vi "XML - Create XML file.vi"(8 "error in (no error)":errorcluster, 10 "Consolidated_CD":refnum<class "NIVS_Consolidated_CDW_MetaDataObj.lvclass">, 11 "CD Wizard - Internal Data":T1) -> (0 "error out":errorcluster)   [LabVIEW 2019, in "NIVS_Consolidated_CDW_MetaDataObj.lvclass"]
doc: "Create the XML file and alter the content of the file, so that it fits for the generated custom device."
uses:
  NIVS_Consolidated_CDW_MetaDataObj.lvclass
  Internal data.ctl
  C:/Program Files (x86)/National Instruments/LabVIEW 2019/resource/dialog/NewProjectWizard/MetaDataObj/MetaDataObj.lvclass
  Create XML-file - States.ctl
  <resource>/dialog/NewProjectWizard/MetaDataObj/MetaDataObj.lvclass/MetaDataObj.ctl
  NIVS_Consolidated_CDW_MetaDataObj.lvclass/NIVS_Consolidated_CDW_MetaDataObj.ctl
  Template Classes/NIVS_CD Template/NIVS_CD Template.lvclass/NIVS_CD Template.ctl
  CD System Explorer lvlib.ctl
  Target Type.ctl
  Template Classes/NIVS_CD Template/Read Submenu.vi
  Template Classes/NIVS_CD Template/Read Parent Menu.vi
  Template Classes/NIVS_CD Template/Read Max Instances.vi
  <resource>/dialog/NewProjectWizard/MetaDataObj/Accessors/Read Project Root.vi
  <resource>/dialog/NewProjectWizard/MetaDataObj/Accessors/Read Project Name.vi
  Read CD Template.vi
  CD System Explorer lvlib.vi
  Template Classes/NIVS_CD Template/NIVS_CD Template.lvclass
  <vilib>/Utility/Data Type/NI_Data Type.lvlib
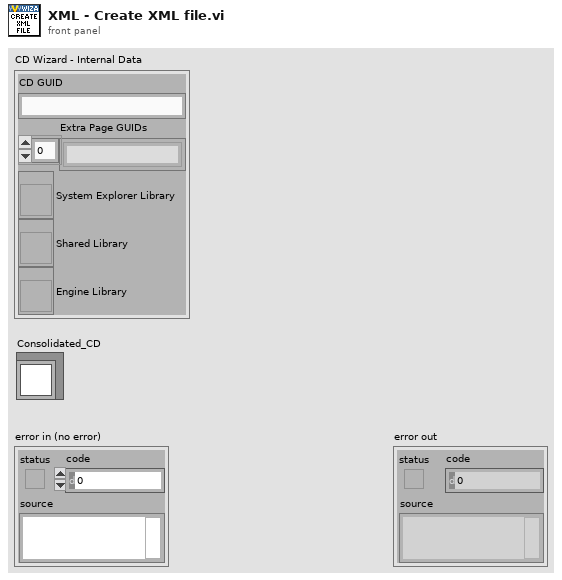
[diagram p1: front panel]
types:
  T1 = typedef "NIVS_Consolidated_CDW_MetaDataObj.lvclass/Internal data.ctl" = cluster{"CD GUID":string, "Extra Page GUIDs":string[], "System Explorer Library":refnum<vi>, "Shared Library":refnum<vi>, "Engine Library":refnum<vi>}
  T2 = typedef "NIVS_Consolidated_CDW_MetaDataObj.lvclass/Create XML-file - States.ctl" = enum16{"Read XML template file", "Change CD -MenuName-", "Change CD -Name-", "Change CD -Type-", "Change CD -Occurrences-", "Change CD -MainPageGUID-", "Change CD -InitVIPath-", "Change CD -WindowsCustomDeviceVIPath-", "Change CD -WindowsCustomDeviceVIRTPath-", "Change CD -PharlapCustomDeviceVIPath-", "Change CD -PharlapCustomDeviceVIRTPath-", "Change CD -VxWorksCustomDeviceVIPath-", "Change CD -VxWorksCustomDeviceVIRTPath-", "Change CD -LinuxARMCustomDeviceVIPath-", "Change CD -LinuxARMCustomDeviceVIRTPath-", "Change CD -Linuxx64CustomDeviceVIPath-", "Change CD -Linuxx64CustomDeviceVIRTPath-", "Change CD -MainPageVIPath-", "Change CD -ExtraPages-", "Change CD -ActionVIOnCompile-", "Change CD -ExportConfigurationRTM-", "Write XML file content back"}
  T3 = typedef "NIVS_Consolidated_CDW_MetaDataObj.lvclass/CD System Explorer lvlib.ctl" = enum16{"LibraryFileName", "LibraryFolderName", "System Explorer.FolderName", "System Explorer.Dynamically Called.FolderName", "System Explorer.Dynamically Called.Extra Pages.FolderName", "System Explorer.Dynamically Called.Extra Pages.TemplatePathAndName", "System Explorer.Dynamically Called.Main Page.VIName", "System Explorer.Dynamically Called.Main Page.TemplatePathAndName", "System Explorer.Dynamically Called.Initialization VI.VIName", "System Explorer.Dynamically Called.Initialization VI.TemplatePathAndName", "System Explorer.SubVI.FolderName", "System Explorer.Types.FolderName", "System Explorer.ActionVIOnCompile.VIName", "System Explorer.ExportConfigRTM.VIName", "System Explorer.LoadHelpFile.VIName"}
  T4 = typedef "NIVS_Consolidated_CDW_MetaDataObj.lvclass/Target Type.ctl" = enum16{"Windows", "VxWorks", "Pharlap", "Linux 32 ARM", "Linux x64"}
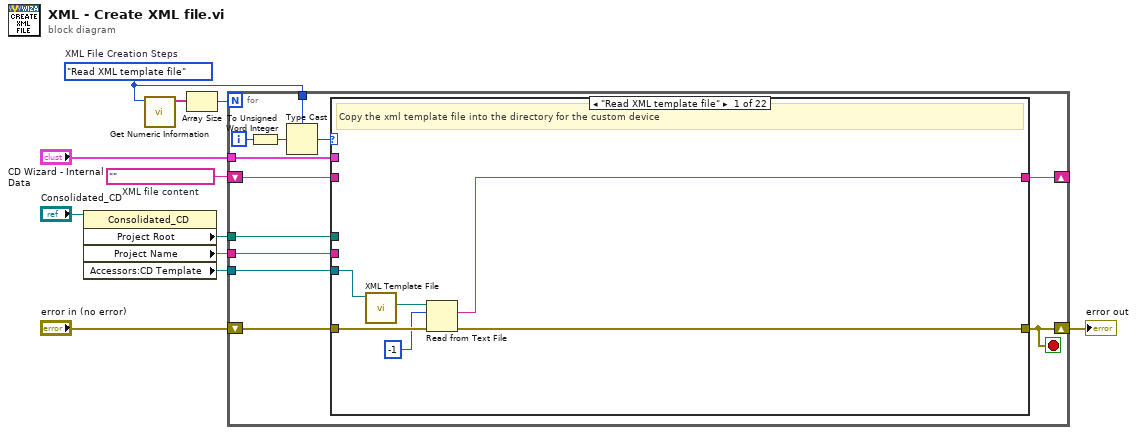
[diagram p0: block diagram]
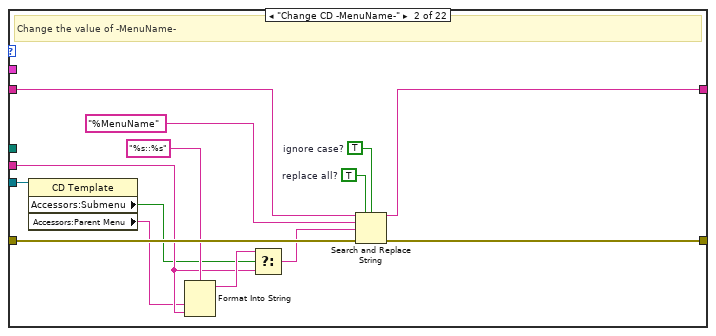
[diagram p2: hidden frame]
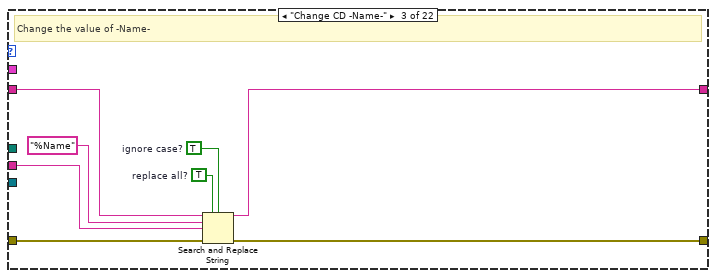
[diagram p3: hidden frame]
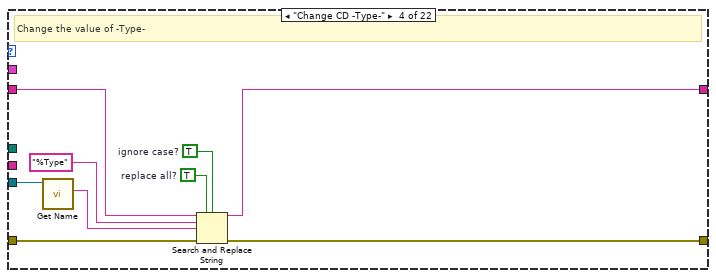
[diagram p4: hidden frame]
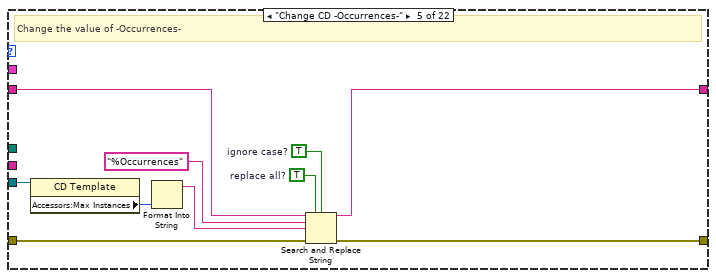
[diagram p5: hidden frame]
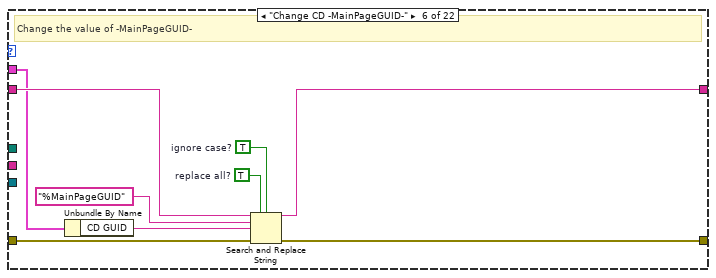
[diagram p6: hidden frame]
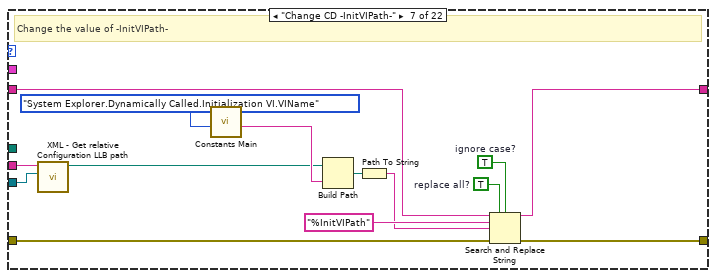
[diagram p7: hidden frame]
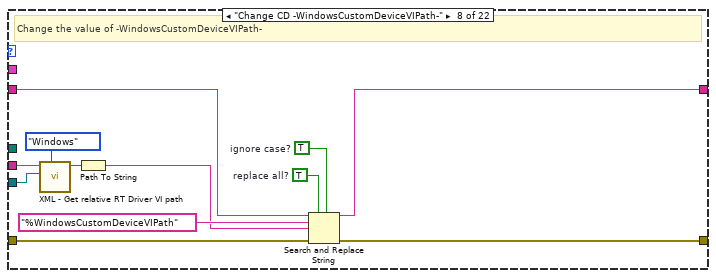
[diagram p8: hidden frame]
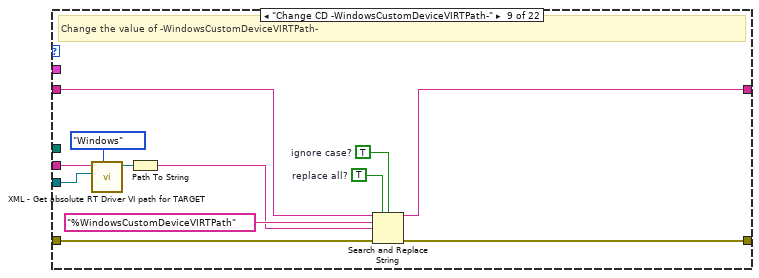
[diagram p9: hidden frame]
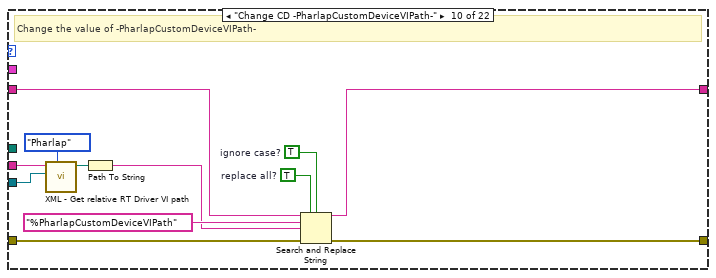
[diagram p10: hidden frame]
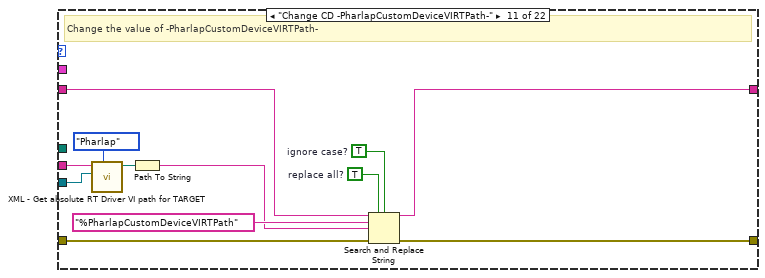
[diagram p11: hidden frame]
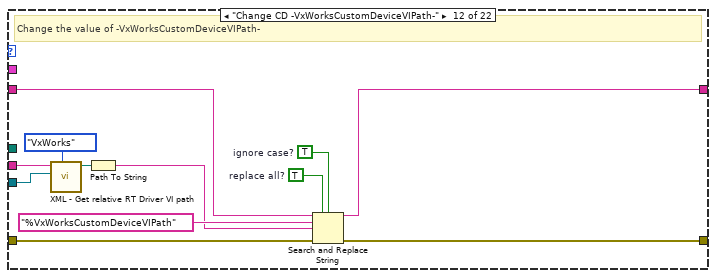
[diagram p12: hidden frame]
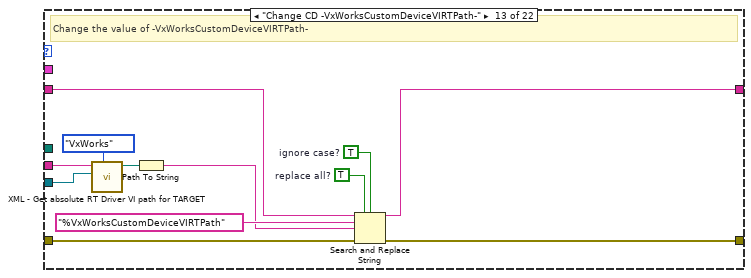
[diagram p13: hidden frame]
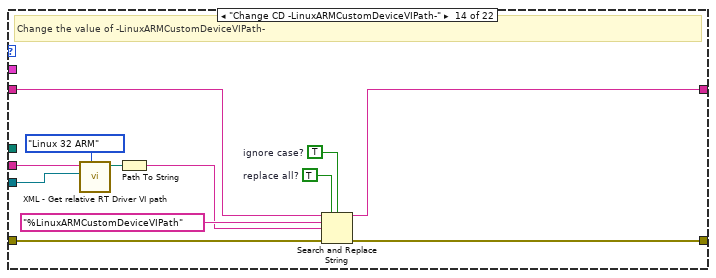
[diagram p14: hidden frame]
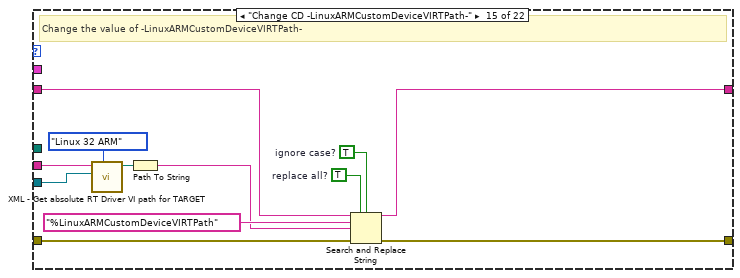
[diagram p15: hidden frame]
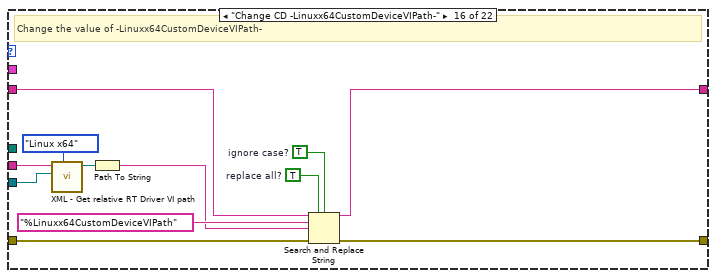
[diagram p16: hidden frame]
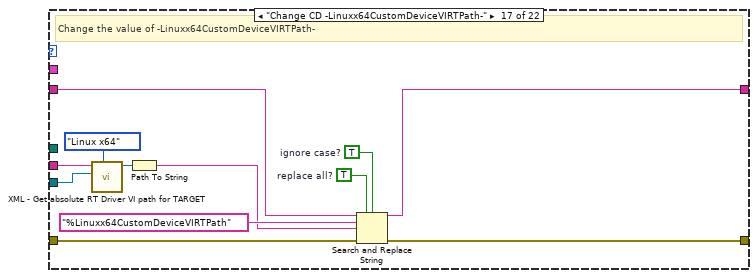
[diagram p17: hidden frame]
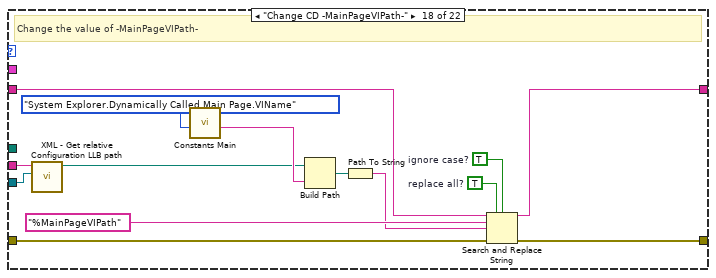
[diagram p18: hidden frame]
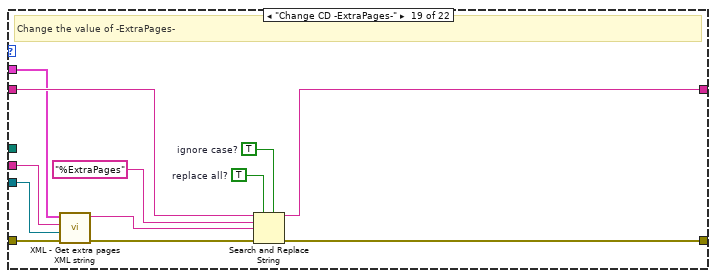
[diagram p19: hidden frame]
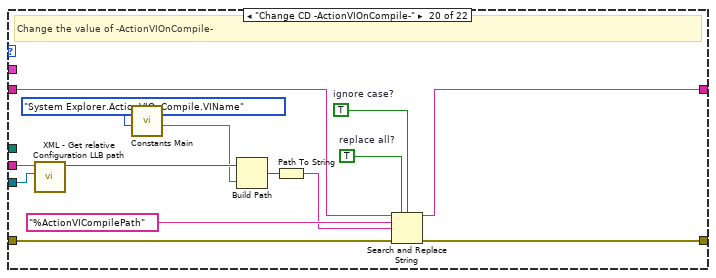
[diagram p20: hidden frame]
diagram:
  w2 = Create_XML-file_-_States."Read XML template file"  # XML File Creation Steps
  w10 = ""  # XML file content
  n1 = property class="Consolidated_CD"(reference="Consolidated_CD") -> ("Project Root"=w8:path, "Project Name"=w7:string, "Accessors:CD Template"=w6:refnum<class "NIVS_CD Template.lvclass">)  [unwired: 1 in, 2 out]
  n2 = call <vilib>:"Get Numeric Information.vi"("variant"=w2) -> ("enum names"=w3:string[])  [unwired: 7 in, 3 out]
  n3 = Array Size(array=w3) -> (size(s)=w4:i32)
  n4 = for {
    N: w4 -> [_]
    shift-right: [w18] -> w11
    shift-left: "error in (no error)" -> [w17]
    shift-right: [w22] -> _
    shift-left: w10 -> [w23]
    tunnel: w8 -> [w21]
    tunnel: w7 -> [w20]
    tunnel: w6 -> [w19]
    tunnel: w2 -> [w15]
    tunnel: "CD Wizard - Internal Data" -> [w12]
    i -> [w16]
    stop <- w18 stop-if-true
    # "While loop for State Machine"
    n5 = To Unsigned Word Integer(number=w16) -> (unsigned 16bit integer=w14:u16)
    n6 = Type Cast(type=w15, x=w14) -> (*(type *) &x=w13:T2)
    n7 = case shown="\"Read XML template file\"" w13 {
      tunnel: w17 -> [w27 w39 w47 w54 w61 w72 w82 w96 w108 w120 w132 w144 w156 w168 w180 w192 w204 w216 w230 w240 w254 w277]
      tunnel: [w28 w40 w48 w57 w67 w76 w90 w104 w115 w127 w139 w151 w163 w175 w187 w199 w211 w224 w236 w250 w257 w280] -> w18
      tunnel: w12 -> [_ _ _ _ _ w75 _ _ _ _ _ _ _ _ _ _ _ _ w234 _ _ _]
      tunnel: w23 -> [_ w42 w50 w59 w69 w78 w92 w101 w117 w129 w141 w153 w165 w177 w189 w201 w213 w226 w238 w252 w271 w279]
      tunnel: [w24 w41 w49 w58 w68 w77 w91 w105 w116 w128 w140 w152 w164 w176 w188 w200 w212 w225 w237 w251 w261 w279] -> w22
      tunnel: w21 -> [_ _ _ _ _ _ _ _ _ _ _ _ _ _ _ _ _ _ _ _ _ w276]
      tunnel: w20 -> [_ w33 w44 _ _ _ w81 w95 w107 w119 w131 w143 w155 w167 w179 w191 w203 w215 w229 w242 w256 w275]
      tunnel: w19 -> [w29 w32 _ w53 w63 _ w80 w94 w106 w118 w130 w142 w154 w166 w178 w190 w202 w214 w228 w241 w255 w274]
      frame "Read XML template file" {
        # "Copy the xml template file into the directory for the custom device"
        n8 = call-dynamic "XML Template File.vi"("CD Template"=w29) -> ("XML Template File"=w26:path)  [unwired: 10 in]
        n9 = Read from Text File(file (use dialog)=w26, count=-1, error in=w27) -> (text=w24:string, error out=w28:errorcluster)  [unwired: 1 in, 2 out]
      }
      frame "Change CD -MenuName-" {
        w37 = TRUE  # ignore case?
        w38 = TRUE  # replace all?
        # "Change the value of -MenuName-"
        n10 = property class="CD Template"(reference=w32) -> ("Accessors:Submenu"=w31:bool, "Accessors:Parent Menu"=w30:string)  [unwired: 1 in, 2 out]
        n11 = Format Into String(format string="%s::%s", w30, w33) -> (resulting string=w35:string)  [unwired: 2 in, 1 out]
        n12 = Select(t=w35, s=w31, f=w33) -> (s? t:f=w34:string)
        n13 = Search and Replace String(replace all?=w38, case sensitive?=w37, input string=w42, search string="%MenuName", replace string=w34, error in=w39) -> (result string=w41:string, error out=w40:errorcluster)  [unwired: 1 in, 3 out]
      }
      frame "Change CD -Name-" {
        w45 = TRUE  # ignore case?
        w46 = TRUE  # replace all?
        # "Change the value of -Name-"
        n14 = Search and Replace String(replace all?=w46, case sensitive?=w45, input string=w50, search string="%Name", replace string=w44, error in=w47) -> (result string=w49:string, error out=w48:errorcluster)  [unwired: 1 in, 3 out]
      }
      frame "Change CD -Type-" {
        w55 = TRUE  # ignore case?
        w56 = TRUE  # replace all?
        # "Change the value of -Type-"
        n15 = call-dynamic "Get Name.vi"("CD Template"=w53) -> ("String"=w52:string)  [unwired: 10 in]
        n16 = Search and Replace String(replace all?=w56, case sensitive?=w55, input string=w59, search string="%Type", replace string=w52, error in=w54) -> (result string=w58:string, error out=w57:errorcluster)  [unwired: 1 in, 3 out]
      }
      frame "Change CD -Occurrences-" {
        w64 = TRUE  # ignore case?
        w66 = TRUE  # replace all?
        # "Change the value of -Occurrences-"
        n17 = property class="CD Template"(reference=w63) -> ("Accessors:Max Instances"=w62:u32)  [unwired: 1 in, 2 out]
        n18 = Format Into String(w62) -> (resulting string=w65:string)  [unwired: 3 in, 1 out]
        n19 = Search and Replace String(replace all?=w66, case sensitive?=w64, input string=w69, search string="%Occurrences", replace string=w65, error in=w61) -> (result string=w68:string, error out=w67:errorcluster)  [unwired: 1 in, 3 out]
      }
      frame "Change CD -MainPageGUID-" {
        w71 = TRUE  # ignore case?
        w74 = TRUE  # replace all?
        # "Change the value of -MainPageGUID-"
        n20 = Unbundle By Name(w75) -> ("CD GUID"=w73:string)
        n21 = Search and Replace String(replace all?=w74, case sensitive?=w71, input string=w78, search string="%MainPageGUID", replace string=w73, error in=w72) -> (result string=w77:string, error out=w76:errorcluster)  [unwired: 1 in, 3 out]
      }
      frame "Change CD -InitVIPath-" {
        w88 = TRUE  # ignore case?
        w89 = TRUE  # replace all?
        # "Change the value of -InitVIPath-"
        n22 = call "XML - Get relative Configuration LLB path.vi"("CD Template"=w80, "Project Name"=w81) -> ("Relative Configuration LLB path"=w83:path)  [unwired: 9 in]
        n23 = call-poly "Constants Main.vi"("Action"=CD_System_Explorer_lvlib."System Explorer.Dynamically Called.Initialization VI.VIName") -> ("Output"=w86:string)  [unwired: 10 in]
        n24 = Build Path(base path=w83, name or relative path=w86) -> (appended path=w84:path)
        n25 = Path To String(path=w84) -> (string=w87:string)
        n26 = Search and Replace String(replace all?=w89, case sensitive?=w88, input string=w92, search string="%InitVIPath", replace string=w87, error in=w82) -> (result string=w91:string, error out=w90:errorcluster)  [unwired: 1 in, 3 out]
      }
      frame "Change CD -WindowsCustomDeviceVIPath-" {
        w102 = TRUE  # ignore case?
        w103 = TRUE  # replace all?
        # "Change the value of -WindowsCustomDeviceVIPath-"
        n27 = call "XML - Get relative RT Driver VI path.vi"("Target Type (Windows)"=Target_Type."Windows", "CD Template"=w94, "Project Name"=w95) -> ("Relative RT Driver VI path"=w97:path)  [unwired: 8 in]
        n28 = Path To String(path=w97) -> (string=w99:string)
        n29 = Search and Replace String(replace all?=w103, case sensitive?=w102, input string=w101, search string="%WindowsCustomDeviceVIPath", replace string=w99, error in=w96) -> (result string=w105:string, error out=w104:errorcluster)  [unwired: 1 in, 3 out]
      }
      frame "Change CD -WindowsCustomDeviceVIRTPath-" {
        w113 = TRUE  # ignore case?
        w114 = TRUE  # replace all?
        # "Change the value of -WindowsCustomDeviceVIRTPath-"
        n30 = call "XML - Get absolute RT Driver VI path for TARGET.vi"("Target Type (Windows)"=Target_Type."Windows", "CD Template"=w106, "Project Name"=w107) -> ("Relative RT Driver TARGET path"=w109:path)  [unwired: 8 in]
        n31 = Path To String(path=w109) -> (string=w111:string)
        n32 = Search and Replace String(replace all?=w114, case sensitive?=w113, input string=w117, search string="%WindowsCustomDeviceVIRTPath", replace string=w111, error in=w108) -> (result string=w116:string, error out=w115:errorcluster)  [unwired: 1 in, 3 out]
      }
      frame "Change CD -PharlapCustomDeviceVIPath-" {
        w125 = TRUE  # ignore case?
        w126 = TRUE  # replace all?
        # "Change the value of -PharlapCustomDeviceVIPath-"
        n33 = call "XML - Get relative RT Driver VI path.vi"("Target Type (Windows)"=Target_Type."Pharlap", "CD Template"=w118, "Project Name"=w119) -> ("Relative RT Driver VI path"=w121:path)  [unwired: 8 in]
        n34 = Path To String(path=w121) -> (string=w122:string)
        n35 = Search and Replace String(replace all?=w126, case sensitive?=w125, input string=w129, search string="%PharlapCustomDeviceVIPath", replace string=w122, error in=w120) -> (result string=w128:string, error out=w127:errorcluster)  [unwired: 1 in, 3 out]
      }
      frame "Change CD -PharlapCustomDeviceVIRTPath-" {
        w137 = TRUE  # ignore case?
        w138 = TRUE  # replace all?
        # "Change the value of -PharlapCustomDeviceVIRTPath-"
        n36 = call "XML - Get absolute RT Driver VI path for TARGET.vi"("Target Type (Windows)"=Target_Type."Pharlap", "CD Template"=w130, "Project Name"=w131) -> ("Relative RT Driver TARGET path"=w133:path)  [unwired: 8 in]
        n37 = Path To String(path=w133) -> (string=w134:string)
        n38 = Search and Replace String(replace all?=w138, case sensitive?=w137, input string=w141, search string="%PharlapCustomDeviceVIRTPath", replace string=w134, error in=w132) -> (result string=w140:string, error out=w139:errorcluster)  [unwired: 1 in, 3 out]
      }
      frame "Change CD -VxWorksCustomDeviceVIPath-" {
        w149 = TRUE  # ignore case?
        w150 = TRUE  # replace all?
        # "Change the value of -VxWorksCustomDeviceVIPath-"
        n39 = call "XML - Get relative RT Driver VI path.vi"("Target Type (Windows)"=Target_Type."VxWorks", "CD Template"=w142, "Project Name"=w143) -> ("Relative RT Driver VI path"=w145:path)  [unwired: 8 in]
        n40 = Path To String(path=w145) -> (string=w146:string)
        n41 = Search and Replace String(replace all?=w150, case sensitive?=w149, input string=w153, search string="%VxWorksCustomDeviceVIPath", replace string=w146, error in=w144) -> (result string=w152:string, error out=w151:errorcluster)  [unwired: 1 in, 3 out]
      }
      frame "Change CD -VxWorksCustomDeviceVIRTPath-" {
        w161 = TRUE  # ignore case?
        w162 = TRUE  # replace all?
        # "Change the value of -VxWorksCustomDeviceVIRTPath-"
        n42 = call "XML - Get absolute RT Driver VI path for TARGET.vi"("Target Type (Windows)"=Target_Type."VxWorks", "CD Template"=w154, "Project Name"=w155) -> ("Relative RT Driver TARGET path"=w157:path)  [unwired: 8 in]
        n43 = Path To String(path=w157) -> (string=w158:string)
        n44 = Search and Replace String(replace all?=w162, case sensitive?=w161, input string=w165, search string="%VxWorksCustomDeviceVIRTPath", replace string=w158, error in=w156) -> (result string=w164:string, error out=w163:errorcluster)  [unwired: 1 in, 3 out]
      }
      frame "Change CD -LinuxARMCustomDeviceVIPath-" {
        w173 = TRUE  # ignore case?
        w174 = TRUE  # replace all?
        # "Change the value of -LinuxARMCustomDeviceVIPath-"
        n45 = call "XML - Get relative RT Driver VI path.vi"("Target Type (Windows)"=Target_Type."Linux 32 ARM", "CD Template"=w166, "Project Name"=w167) -> ("Relative RT Driver VI path"=w169:path)  [unwired: 8 in]
        n46 = Path To String(path=w169) -> (string=w171:string)
        n47 = Search and Replace String(replace all?=w174, case sensitive?=w173, input string=w177, search string="%LinuxARMCustomDeviceVIPath", replace string=w171, error in=w168) -> (result string=w176:string, error out=w175:errorcluster)  [unwired: 1 in, 3 out]
      }
      frame "Change CD -LinuxARMCustomDeviceVIRTPath-" {
        w185 = TRUE  # ignore case?
        w186 = TRUE  # replace all?
        # "Change the value of -LinuxARMCustomDeviceVIRTPath-"
        n48 = call "XML - Get absolute RT Driver VI path for TARGET.vi"("Target Type (Windows)"=Target_Type."Linux 32 ARM", "CD Template"=w178, "Project Name"=w179) -> ("Relative RT Driver TARGET path"=w181:path)  [unwired: 8 in]
        n49 = Path To String(path=w181) -> (string=w182:string)
        n50 = Search and Replace String(replace all?=w186, case sensitive?=w185, input string=w189, search string="%LinuxARMCustomDeviceVIRTPath", replace string=w182, error in=w180) -> (result string=w188:string, error out=w187:errorcluster)  [unwired: 1 in, 3 out]
      }
      frame "Change CD -Linuxx64CustomDeviceVIPath-" {
        w197 = TRUE  # ignore case?
        w198 = TRUE  # replace all?
        # "Change the value of -Linuxx64CustomDeviceVIPath-"
        n51 = call "XML - Get relative RT Driver VI path.vi"("Target Type (Windows)"=Target_Type."Linux x64", "CD Template"=w190, "Project Name"=w191) -> ("Relative RT Driver VI path"=w193:path)  [unwired: 8 in]
        n52 = Path To String(path=w193) -> (string=w195:string)
        n53 = Search and Replace String(replace all?=w198, case sensitive?=w197, input string=w201, search string="%Linuxx64CustomDeviceVIPath", replace string=w195, error in=w192) -> (result string=w200:string, error out=w199:errorcluster)  [unwired: 1 in, 3 out]
      }
      frame "Change CD -Linuxx64CustomDeviceVIRTPath-" {
        w209 = TRUE  # ignore case?
        w210 = TRUE  # replace all?
        # "Change the value of -Linuxx64CustomDeviceVIRTPath-"
        n54 = call "XML - Get absolute RT Driver VI path for TARGET.vi"("Target Type (Windows)"=Target_Type."Linux x64", "CD Template"=w202, "Project Name"=w203) -> ("Relative RT Driver TARGET path"=w205:path)  [unwired: 8 in]
        n55 = Path To String(path=w205) -> (string=w206:string)
        n56 = Search and Replace String(replace all?=w210, case sensitive?=w209, input string=w213, search string="%Linuxx64CustomDeviceVIRTPath", replace string=w206, error in=w204) -> (result string=w212:string, error out=w211:errorcluster)  [unwired: 1 in, 3 out]
      }
      frame "Change CD -MainPageVIPath-" {
        w222 = TRUE  # ignore case?
        w223 = TRUE  # replace all?
        # "Change the value of -MainPageVIPath-"
        n57 = call "XML - Get relative Configuration LLB path.vi"("CD Template"=w214, "Project Name"=w215) -> ("Relative Configuration LLB path"=w217:path)  [unwired: 9 in]
        n58 = call-poly "Constants Main.vi"("Action"=CD_System_Explorer_lvlib."System Explorer.Dynamically Called.Main Page.VIName") -> ("Output"=w221:string)  [unwired: 10 in]
        n59 = Build Path(base path=w217, name or relative path=w221) -> (appended path=w219:path)
        n60 = Path To String(path=w219) -> (string=w218:string)
        n61 = Search and Replace String(replace all?=w223, case sensitive?=w222, input string=w226, search string="%MainPageVIPath", replace string=w218, error in=w216) -> (result string=w225:string, error out=w224:errorcluster)  [unwired: 1 in, 3 out]
      }
      frame "Change CD -ExtraPages-" {
        w232 = TRUE  # ignore case?
        w235 = TRUE  # replace all?
        # "Change the value of -ExtraPages-"
        n62 = call "XML - Get extra pages XML string.vi"("error in (no error)"=w230, "CD Template"=w228, "Project Name"=w229, "CD Wizard - Internal Data"=w234) -> ("error out"=w231:errorcluster, "Extra Pages XML string"=w233:string)  [unwired: 6 in]
        n63 = Search and Replace String(replace all?=w235, case sensitive?=w232, input string=w238, search string="%ExtraPages", replace string=w233, error in=w231) -> (result string=w237:string, error out=w236:errorcluster)  [unwired: 1 in, 3 out]
      }
      frame "Change CD -ActionVIOnCompile-" {
        w248 = TRUE  # ignore case?
        w249 = TRUE  # replace all?
        # "Change the value of -ActionVIOnCompile-"
        n64 = call "XML - Get relative Configuration LLB path.vi"("CD Template"=w241, "Project Name"=w242) -> ("Relative Configuration LLB path"=w247:path)  [unwired: 9 in]
        n65 = call-poly "Constants Main.vi"("Action"=CD_System_Explorer_lvlib."System Explorer.ActionVIOnCompile.VIName") -> ("Output"=w243:string)  [unwired: 10 in]
        n66 = Build Path(base path=w247, name or relative path=w243) -> (appended path=w246:path)
        n67 = Path To String(path=w246) -> (string=w245:string)
        n68 = Search and Replace String(replace all?=w249, case sensitive?=w248, input string=w252, search string="%ActionVICompilePath", replace string=w245, error in=w240) -> (result string=w251:string, error out=w250:errorcluster)  [unwired: 1 in, 3 out]
      }
      frame "Change CD -ExportConfigurationRTM-" {
        w264 = TRUE  # ignore case?
        w263 = TRUE  # replace all?
        # "Change the value of -ExportConfigurationRTM-"
        n69 = call "XML - Get relative Configuration LLB path.vi"("CD Template"=w255, "Project Name"=w256) -> ("Relative Configuration LLB path"=w270:path)  [unwired: 9 in]
        n70 = call-poly "Constants Main.vi"("Action"=CD_System_Explorer_lvlib."System Explorer.ExportConfigRTM.VIName") -> ("Output"=w266:string)  [unwired: 10 in]
        n71 = Build Path(base path=w270, name or relative path=w266) -> (appended path=w269:path)
        n72 = Path To String(path=w269) -> (string=w268:string)
        n73 = Search and Replace String(replace all?=w263, case sensitive?=w264, input string=w271, search string="%ExportConfigurationRTMPath", replace string=w268, error in=w254) -> (result string=w262:string, error out=w260:errorcluster)  [unwired: 1 in, 3 out]
        n74 = call "Create GUID.vi"("error in (no error)"=w260) -> ("error out"=w258:errorcluster, "Generated GUID"=w259:string)  [unwired: 9 in]
        n75 = Search and Replace String(replace all?=w263, case sensitive?=w264, input string=w262, search string="%ExportConfigurationGUID", replace string=w259, error in=w258) -> (result string=w261:string, error out=w257:errorcluster)  [unwired: 1 in, 3 out]
      }
      frame "Write XML file content back" {
        # "Write the modified file content back to the XML file"
        n76 = call "XML - Get XML file name.vi"("CD Template"=w274, "CD Name"=w275) -> ("XML file name"=w278:string)  [unwired: 9 in]
        n77 = Build Path(base path=w276, name or relative path=w278) -> (appended path=w273:path)
        n78 = Write to Text File(file (use dialog)=w273, text=w279, error in=w277) -> (error out=w280:errorcluster)  [unwired: 3 out]
      }
    }
  }
  "error out" <- w11
